vi "csv_control _01.vi"() -> ()   [LabVIEW 2024]
panel:
  in  "Test_Value":dbl
  in  "Test_ID":string
  in  "SN":string
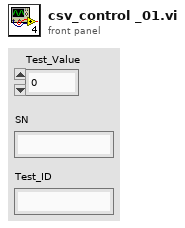
[diagram p1: front panel]
types:
  T1 = enum16{"open", "replace", "create", "open or create", "replace or create", "replace or create with confirmation"}
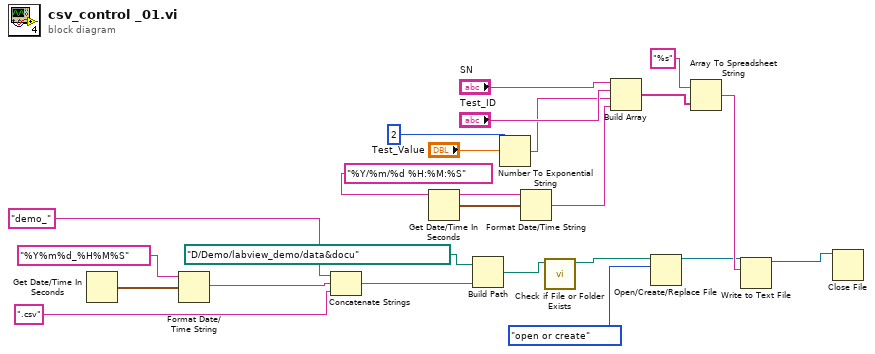
[diagram p0: block diagram]
diagram:
  n1 = Get Date/Time In Seconds() -> (seconds since 1Jan1904=w3:timestamp)
  n2 = Format Date/Time String(time format string (%c)="%Y%m%d_%H%M%S" ("时间格式字符串(%c)"), seconds (now)=w3) -> (date/time string=w1:string)  [unwired: 1 in]
  n3 = Concatenate Strings("demo_" ("字符串"), w1, ".csv" ("字符串")) -> (w5:string)
  n4 = Get Date/Time In Seconds() -> (seconds since 1Jan1904=w17:timestamp)
  n5 = Build Path(base path=path "D:/Demo/labview_demo/data&docu" ("基路径"), name or relative path=w5) -> (appended path=w23:path)
  n6 = Number To Exponential String(number="Test_Value", precision (6)=i16 2 ("精度(6)")) -> (E-format string=w18:string)  [unwired: 2 in]
  n7 = Format Date/Time String(time format string (%c)="%Y/%m/%d %H:%M:%S" ("时间格式字符串(%c)"), seconds (now)=w17) -> (date/time string=w7:string)  [unwired: 1 in]
  n8 = call <vilib>:"Check if File or Folder Exists.vi"("path"=w23) -> ("dup path"=w22:path)  [unwired: 8 in, 2 out]
  n9 = Build Array("SN", "Test_ID", w18, w7) -> (w15:string[])
  n10 = Open/Create/Replace File(file path (use dialog)=w22, operation (0:open)=T1."open or create" ("操作(0:open)")) -> (refnum out=w12:refnum<file>)  [unwired: 4 in, 2 out]
  n11 = Array To Spreadsheet String(array=w15, 3:"%s" ("格式字符串")) -> (spreadsheet string=w14:string)  [unwired: 1 in]
  n12 = Write to Text File(file (use dialog)=w12, text=w14) -> (refnum out=w11:refnum<file>)  [unwired: 2 in, 2 out]
  n13 = Close File(refnum=w11) -> ()  [unwired: 1 in, 2 out]
